vi "4145 Display Graphics.vi"(0 "4145_GPIB_COM_IN":T1={"Address_string"="17", "timeout ms"=25000, "Terminator"=",", "LoggerQueue"=refnum}, 5 "4145_X_Axis_IN":T4={"X axis"=TRUE, "X channel name"="V3", "X scale"=TRUE, "X min"=0.0, "X max"=1.0, "Is X axis VAR 1?"=FALSE} {"X max" format="%^.3e"; "X min" format="%^.3e"}, 7 "4145_Y2_Axis_IN":T2={"Y2 axis"=FALSE, "Y2 channel name"="", "Y2 scale"=TRUE, "Y2 min"=0.0, "Y2 max"=0.01, "# of steps for VAR 2"=0} {"Y2 max" format="%^.3e"; "Y2 min" format="%^.3e"}, 9 "4145_Y_Axis_IN":T3={"Y1 channel name"="I3", "Y1 scale"=TRUE, "Y1 min"=0.0, "Y1 max"=0.01} {"Y1 max" format="%^.3e"; "Y1 min" format="%^.3e"}, 11 "error in":T5) -> (4 "4145_GPIB_COM_OUT":T1={"Address_string"="17", "timeout ms"=25000, "Terminator"=",", "LoggerQueue"=refnum}, 15 "error out":T5)   [LabVIEW 2014]
doc: "This VI sets up the instrument for GRAPHICS mode and configures the X axis, Y1 axis, and Y2 axis."
uses:
  typedef/4145_X_Axis.ctl
  typedef/4145_Y_Axis.ctl
  typedef/4145_Y2_Axis.ctl
  typedef/4145_GPIB_Com.ctl
  typedef/4145_que_msg.ctl
  typedef/4145 command enum.ctl
panel:
  out "concatenated string":string
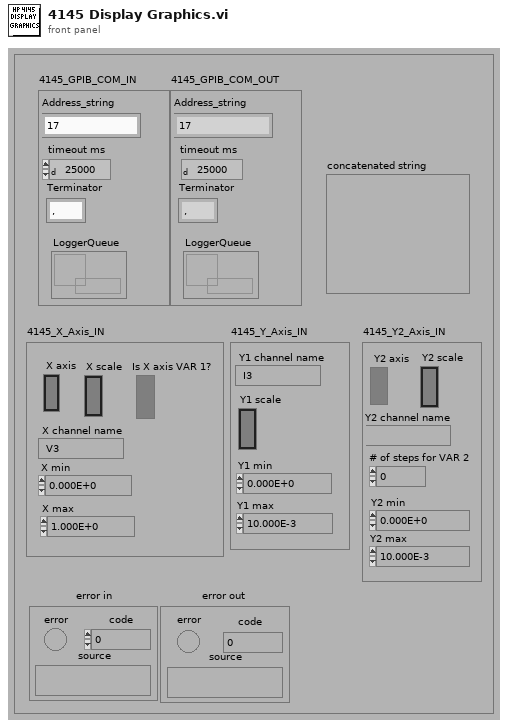
[diagram p1: front panel]
types:
  T1 = typedef "4145_GPIB_Com.ctl" = cluster{"Address_string":string, "timeout ms":u32, "Terminator":string, "LoggerQueue":refnum<queue>}
  T2 = typedef "4145_Y2_Axis.ctl" = cluster{"Y2 axis":bool, "Y2 channel name":string, "Y2 scale":bool, "Y2 min":dbl, "Y2 max":dbl, "# of steps for VAR 2":u16}
  T3 = typedef "4145_Y_Axis.ctl" = cluster{"Y1 channel name":string, "Y1 scale":bool, "Y1 min":dbl, "Y1 max":dbl}
  T4 = typedef "4145_X_Axis.ctl" = cluster{"X axis":bool, "X channel name":string, "X scale":bool, "X min":dbl, "X max":dbl, "Is X axis VAR 1?":bool}
  T5 = cluster{"error":bool, "code":i32, "source":string}
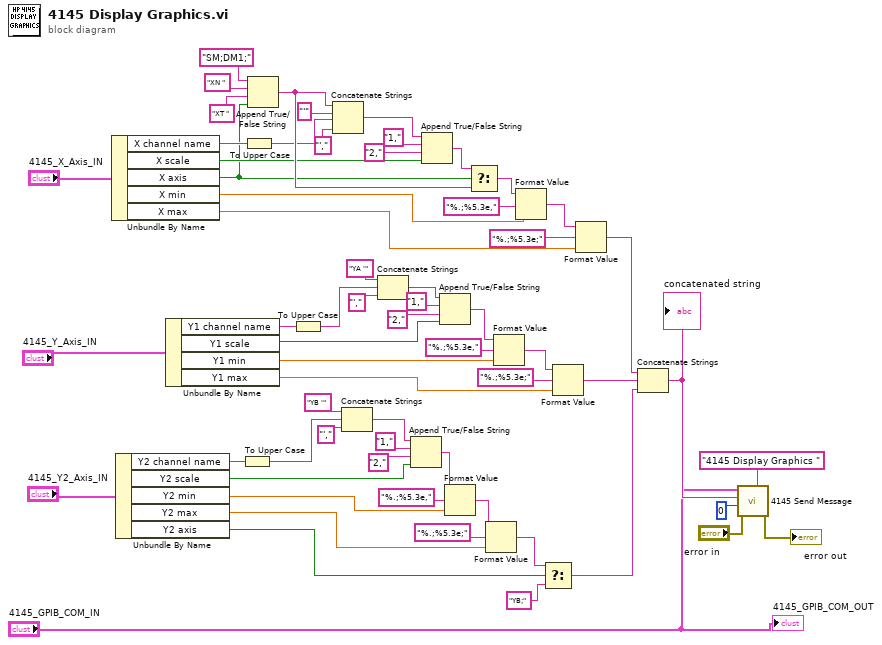
[diagram p0: block diagram]
diagram:
  n1 = Unbundle By Name("4145_X_Axis_IN") -> ("X channel name"=w16:string, "X scale"=w15:bool, "X axis"=w14:bool, "X min"=w13:dbl, "X max"=w12:dbl)
  n2 = Unbundle By Name("4145_Y2_Axis_IN") -> ("Y2 channel name"=w21:string, "Y2 scale"=w20:bool, "Y2 min"=w19:dbl, "Y2 max"=w18:dbl, "Y2 axis"=w17:bool)
  n3 = Unbundle By Name("4145_Y_Axis_IN") -> ("Y1 channel name"=w25:string, "Y1 scale"=w24:bool, "Y1 min"=w23:dbl, "Y1 max"=w22:dbl)
  n4 = To Upper Case(1:w21) -> (0:w6:string)
  n5 = To Upper Case(1:w16) -> (0:w5:string)
  n6 = Append True/False String(1:w14, 2:"XT ", 3:"XN ", 4:"SM;DM1;") -> (0:w54:string)
  n7 = To Upper Case(1:w25) -> (0:w4:string)
  n8 = Concatenate Strings(w54, "'", w5, "',") -> (w59:string)
  n9 = Concatenate Strings("YB '", w6, "',") -> (w38:string)
  n10 = Concatenate Strings("YA '", w4, "',") -> (w45:string)
  n11 = Append True/False String(1:w20, 2:"2,", 3:"1,", 4:w38) -> (0:w32:string)
  n12 = Append True/False String(1:w15, 2:"2,", 3:"1,", 4:w59) -> (0:w55:string)
  n13 = Append True/False String(1:w24, 2:"2,", 3:"1,", 4:w45) -> (0:w41:string)
  n14 = Format Value(string ("")=w32, format string="%.;%5.3e,", value (0)=w19) -> (output string=w35:string)
  n15 = Select(t=w55, s=w14, f=w54) -> (s? t:f=w53:string)
  n16 = Format Value(string ("")=w35, format string="%.;%5.3e;", value (0)=w18) -> (output string=w31:string)
  n17 = Format Value(string ("")=w41, format string="%.;%5.3e,", value (0)=w23) -> (output string=w42:string)
  n18 = Format Value(string ("")=w53, format string="%.;%5.3e,", value (0)=w13) -> (output string=w52:string)
  n19 = Select(t=w31, s=w17, f="YB;") -> (s? t:f=w2:string)
  n20 = Format Value(string ("")=w42, format string="%.;%5.3e;", value (0)=w22) -> (output string=w1:string)
  n21 = Format Value(string ("")=w52, format string="%.;%5.3e;", value (0)=w12) -> (output string=w30:string)
  n22 = Concatenate Strings(w30, w1, w2) -> (w29:string)
  "concatenated string" <- w29
  n23 = call "4145 Send Message.vi"("source IN"="4145 Display Graphics ", "error in"="error in", "write mode (set END:0)"=0, "write buffer IN"=w29, "4145_GPIB_COM_IN"="4145_GPIB_COM_IN") -> ("error out"=→"error out":T5)  [unwired: 3 in, 3 out]
  "4145_GPIB_COM_OUT" <- "4145_GPIB_COM_IN"
